vi "Calc - TEGT Meas.vi"(11 "01-02-9213":dbl[](array[numeric])) -> (3 "TEGT Meas":dbl format="%0.2f")   [LabVIEW 2018, in "Controller (Host).lvlib"]
uses:
  Controller (Host).lvlib
  <vilib>/Analysis/baseanly.llb/Mean (DBL).vi
  <vilib>/Analysis/NI_AALBase.lvlib
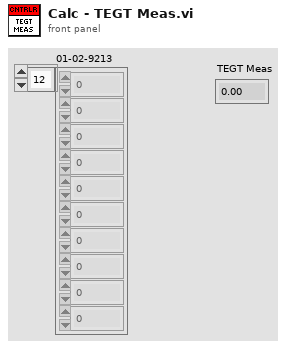
[diagram p1: front panel]
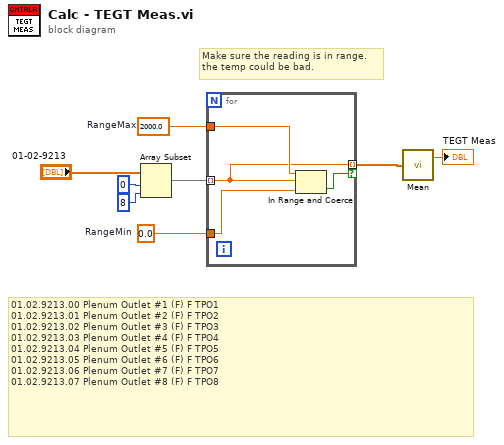
[diagram p0: block diagram]
diagram:
  w3 = 2000.0  # RangeMax
  w4 = 0.0  # RangeMin
  # "01.02.9213.00\tPlenum Outlet #1 (F)\tF\tTPO1\n01.02.9213.01\tPlenum Outlet #2 (F)\tF\tTPO2\n01.02.9213.02\tPlenum Outlet #3 (F)\tF\tTPO3\n01.02.9213.03\tPlenum Outlet #4 (F)\tF\tTPO4\n01.02.9213.04\tPlenum Outlet #5 (F)\tF\tTPO5\n01.02.9213.05\tPlenum Outlet #6 (F)\tF\tTPO6\n01.02.9213.06\tPlenum Outlet #7 (F)\tF\tTPO7\n01.02.9213.07\tPlenum Outlet #8 (F)\tF\tTPO8"
  # "Make sure the reading is in range. \nthe temp could be bad."
  n1 = Array Subset(array="01-02-9213", index=0, length=8) -> (w5:dbl[])
  n2 = for {
    tunnel: w5 -> [w10] mode=indexing
    tunnel: w4 -> [w11]
    tunnel: w3 -> [w12]
    tunnel: [w10] -> w2 mode=indexing if=w9
    n3 = In Range and Coerce(upper limit=w12, x=w10, lower limit=w11) -> (In Range?=w9:bool)  [unwired: 1 out]
  }
  n4 = call-poly <vilib>:"Mean.vi"("X"=w2) -> ("mean"=→"TEGT Meas":dbl)  [unwired: 1 out]
